vi "templates TESTS data keys.vi"(7 "HTM Keys":T1, 8 "error in (no error)":errorcluster, 11 "Connection Refnum":T2) -> (0 "error out":errorcluster, 3 "Connection Refnum":T2, 5 "HTM Keys":T1)   [LabVIEW 2011]
uses:
  Addons/internet/utils/keyedarr.llb/Keyed Array.ctl
  SI.LIB/ODBC/SQL Controls/Connection Refnum.ctl
  Addons/internet/utils/strutil.llb/Case Matching.ctl
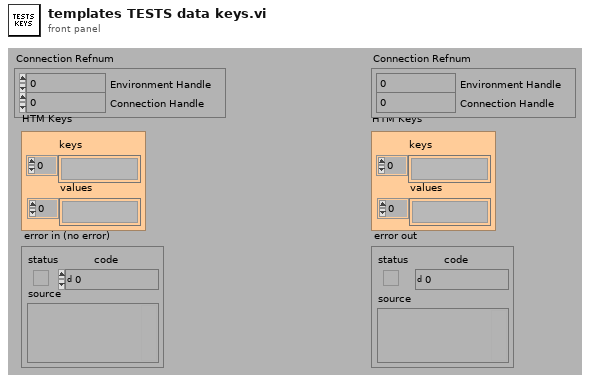
[diagram p1: front panel]
types:
  T1 = typedef "Keyed Array.ctl" = cluster{"keys":string[], "values":string[]}
  T2 = typedef "Connection Refnum.ctl" = cluster{"Environment Handle":i32, "Connection Handle":i32}
  T3 = typedef "Case Matching.ctl" = enum16{"a != A", "a == A", "system"}
  T4 = typedef "Test Record.ctl" = cluster{"ixTest":i32, "sxTestId":string, "sVersion":string, "sDriverTypes":string[], "sDescription":string, "iQuickMode":i32}
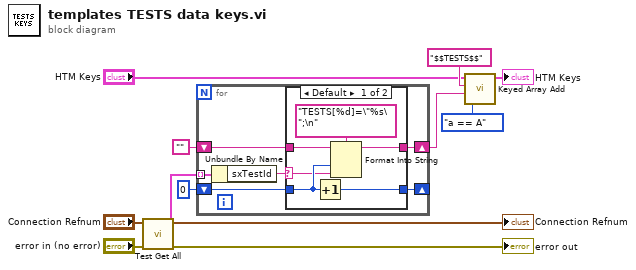
[diagram p0: block diagram]
diagram:
  n1 = call "Test Get All.vi"("error in (no error)"="error in (no error)", "Connection Refnum"="Connection Refnum") -> ("error out"=→"error out":errorcluster, "Test Records"=w12:T4[], "Connection Refnum"=→"Connection Refnum":T2)  [unwired: 2 in, 5 out]
  n2 = for {
    tunnel: w12 -> [w18] mode=indexing
    shift-right: [w16] -> w4
    shift-left: "" -> [w17]
    shift-right: [w13] -> _
    shift-left: 0 -> [w14]
    n3 = Unbundle By Name(w18) -> ("sxTestId"=w15:string)
    n4 = case shown="Default" w15 {
      selector: w15 -> [w20 _]
      tunnel: w17 -> [w24 w26]
      tunnel: [w23 w26] -> w16
      tunnel: w14 -> [w21 w25]
      tunnel: [w22 w25] -> w13
      frame Default {
        n5 = Increment(x=w21) -> (x+1=w22:i32)
        n6 = Format Into String(format string="TESTS[%d]=\"%s\";\n", initial string=w24, w21, w20) -> (resulting string=w23:string)  [unwired: 1 in, 1 out]
      }
      frame "Prompt" {
      }
    }
  }
  n7 = call "Keyed Array Add.vi"("case matching (sensitive)"=Case_Matching."a == A", "value"=w4, "key"="$$TESTS$$", "array in"="HTM Keys") -> ("array out"=→"HTM Keys":T1)  [unwired: 3 out]
